vi "Callback - Shutdown.vi"(8 "error in (no error)":errorcluster, 11 "BluePlotHandleDemo in":refnum<class "NIringPlotHandle.lvclass">) -> (0 "error out":errorcluster, 3 "BluePlotHandleDemo out":refnum<class "NIringPlotHandle.lvclass">)   [LabVIEW 2021, in "NIringPlotHandle.lvclass"]
uses:
  NIringPlotHandle.lvclass
  NIringPlotHandle.lvclass/NIringPlotHandle.ctl
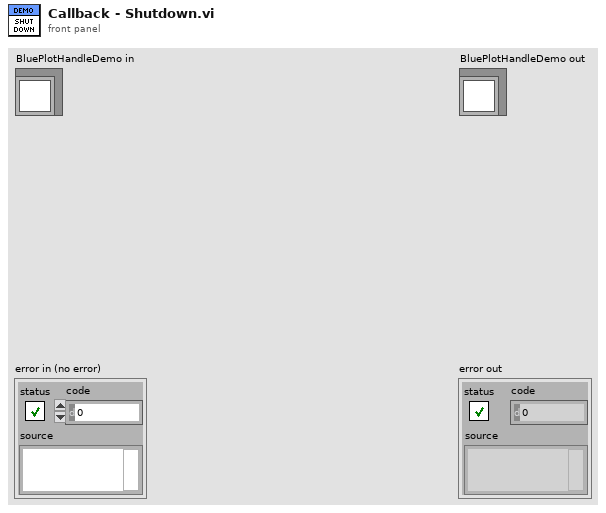
[diagram p1: front panel]
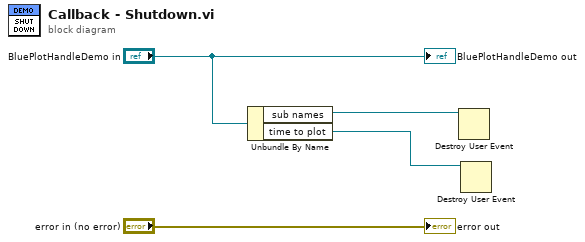
[diagram p0: block diagram]
diagram:
  n1 = Unbundle By Name("BluePlotHandleDemo in") -> ("sub names"=w3:refnum<user-event>, "time to plot"=w2:refnum<user-event>)
  n2 = Destroy User Event(user event=w3) -> ()  [unwired: 1 in, 1 out]
  n3 = Destroy User Event(user event=w2) -> ()  [unwired: 1 in, 1 out]
  "error out" <- "error in (no error)"
  "BluePlotHandleDemo out" <- "BluePlotHandleDemo in"
